vi "pmu_Get Nearest Next Reporting Time.vi"(8 "error in (no error)":errorcluster, 10 "reporting rate":dbl=10.0, 11 "time in":timestamp format="%<%.9X\n%x>T") -> (0 "error out":errorcluster, 3 "reporting time":timestamp format="%<%.9X\n%x>T")   [LabVIEW 2011, in "NI_EP_PMU.lvlib"]
doc: "This VI returns nearest reporting time from the supplied time. The timestamps are aligned so that there is always a reporting time at XX.000 seconds."
uses:
  <vilib>/addons/Electrical Power/PMU/NI_EP_PMU.lvlib
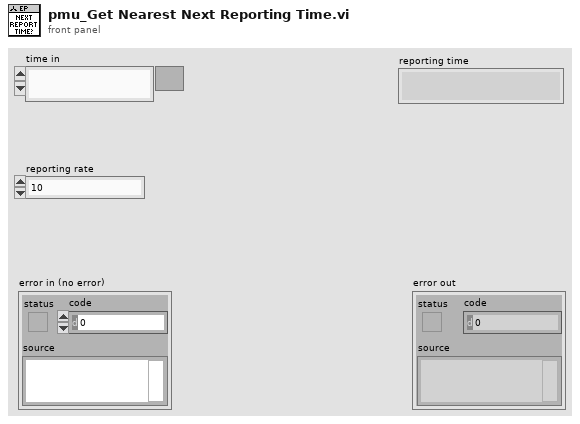
[diagram p1: front panel]
types:
  T1 = typedef "LVDateTimeRec.ctl" = cluster{"fractional second":dbl, "second":i32, "minute":i32, "hour":i32, "day of month":i32, "month":i32, "year":i32, "day of week":i32, "day of year":i32, "DST":i32}
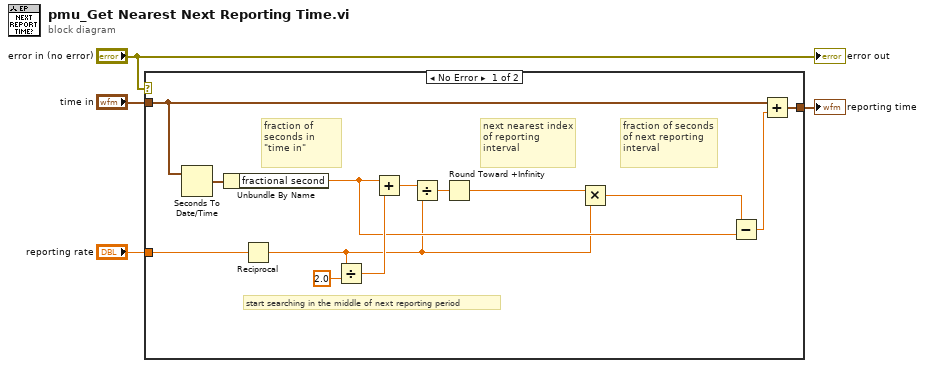
[diagram p0: block diagram]
diagram:
  n1 = case shown="No Error" "error in (no error)" {
    tunnel: "reporting rate" -> [w17 _]
    tunnel: [w15 _] -> w3
    tunnel: "time in" -> [w9 _]
    frame No Error {
      # "start searching in the middle of next reporting period"
      # "fraction of seconds of next reporting interval"
      # "fraction of seconds in \"time in\""
      # "next nearest index of reporting interval"
      n2 = Seconds To Date/Time(time stamp (now)=w9) -> (date time rec=w8:T1)  [unwired: 1 in]
      n3 = Unbundle By Name(w8) -> ("fractional second"=w7:dbl)
      n4 = Reciprocal(x=w17) -> (1/x=w5:dbl)
      n5 = Divide(x=w5, y=2.0) -> (x/y=w11:dbl)
      n6 = Add(x=w7, y=w11) -> (x+y=w13:dbl)
      n7 = Divide(x=w13, y=w5) -> (x/y=w14:dbl)
      n8 = Round Toward +Infinity(x=w14) -> (ceil(x): smallest int >= x=w16:dbl)
      n9 = Multiply(x=w16, y=w5) -> (x*y=w6:dbl)
      n10 = Subtract(x=w6, y=w7) -> (x-y=w10:dbl)
      n11 = Add(x=w9, y=w10) -> (x+y=w15:timestamp)
    }
    frame Error {
    }
  }
  "reporting time" <- w3
  "error out" <- "error in (no error)"
